vi "Synth Power Up.vi"(8 "Error In":errorcluster, 11 "DAQmx Device Name":tag) -> (0 "Error Out":errorcluster, 3 "DAQmx Device Name out":tag)   [LabVIEW 2015]
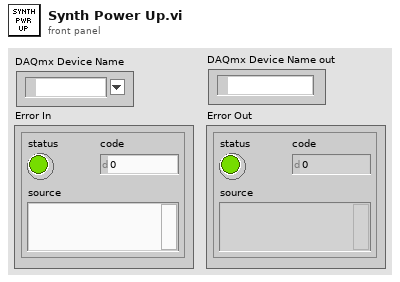
[diagram p1: front panel]
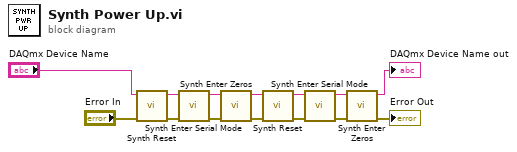
[diagram p0: block diagram]
diagram:
  n1 = call "Synth Reset.vi"("Error In"="Error In", "DAQmx Device Name"="DAQmx Device Name") -> ("Error Out"=w13:errorcluster, "DAQmx Device Name out"=w11:tag)  [unwired: 8 in]
  n2 = call "Synth Enter Serial Mode.vi"("Error In"=w13, "DAQmx Device Name"=w11) -> ("Error Out"=w14:errorcluster, "DAQmx Device Name out"=w10:tag)  [unwired: 8 in]
  n3 = call "Synth Enter Zeros.vi"("Error In"=w14, "DAQmx Device Name"=w10) -> ("Error Out"=w5:errorcluster, "DAQmx Device Name out"=w4:tag)  [unwired: 8 in]
  n4 = call "Synth Reset.vi"("Error In"=w5, "DAQmx Device Name"=w4) -> ("Error Out"=w7:errorcluster, "DAQmx Device Name out"=w8:tag)  [unwired: 8 in]
  n5 = call "Synth Enter Serial Mode.vi"("Error In"=w7, "DAQmx Device Name"=w8) -> ("Error Out"=w6:errorcluster, "DAQmx Device Name out"=w9:tag)  [unwired: 8 in]
  n6 = call "Synth Enter Zeros.vi"("Error In"=w6, "DAQmx Device Name"=w9) -> ("Error Out"=→"Error Out":errorcluster, "DAQmx Device Name out"=→"DAQmx Device Name out":tag)  [unwired: 8 in]
